vi "Configure Overvoltage protection.vi"(8 "error":errorcluster, 10 "OVP Level":dbl format="%.4f", 11 "VISA in":refnum<visa-resource-name>) -> (0 "error out":errorcluster, 3 "VISA out":refnum<visa-resource-name>)   [LabVIEW 2023, in "TDK20-38 API.lvlib"]
uses:
  TDK20-38 API.lvlib
  LabVIEW - Drivers/Genesys Drivers/LAN/TDK-Lambda GEN LAN Series.lvlib
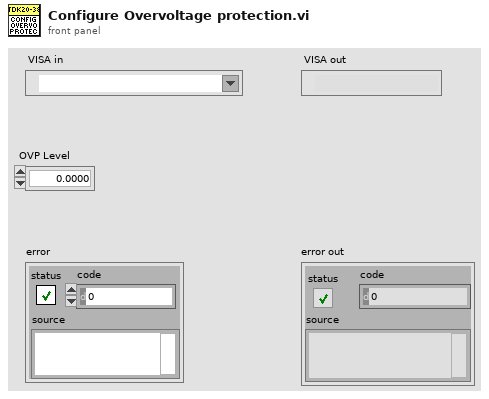
[diagram p1: front panel]
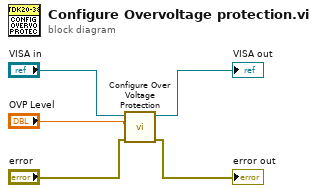
[diagram p0: block diagram]
diagram:
  n1 = call "Configure Over Voltage Protection.vi"("error"="error", "OVP Level"="OVP Level", "VISA"="VISA in") -> ("error out"=→"error out":errorcluster, "VISA out"=→"VISA out":refnum<visa-resource-name>)  [unwired: 7 in]
